vi "Open measure - MAIN.vi"() -> ()   [LabVIEW 2019]
uses:
  OPEN STATUS.ctl
  Open measure - global.vi
panel:
  in  "Normalize":bool
  in  "Remove baseline":bool
  in  "Export image":bool
  out "Phase":cluster{"all rows":dbl[], "all rows":dbl[]}[](graph)
  in  "Add Button":bool
  in  "Clear":bool
  in  "Stop Button":bool
  in  "Plot_name (if only one)":string
  out "Amplitude":cluster{"all rows":dbl[], "all rows":dbl[]}[](graph)
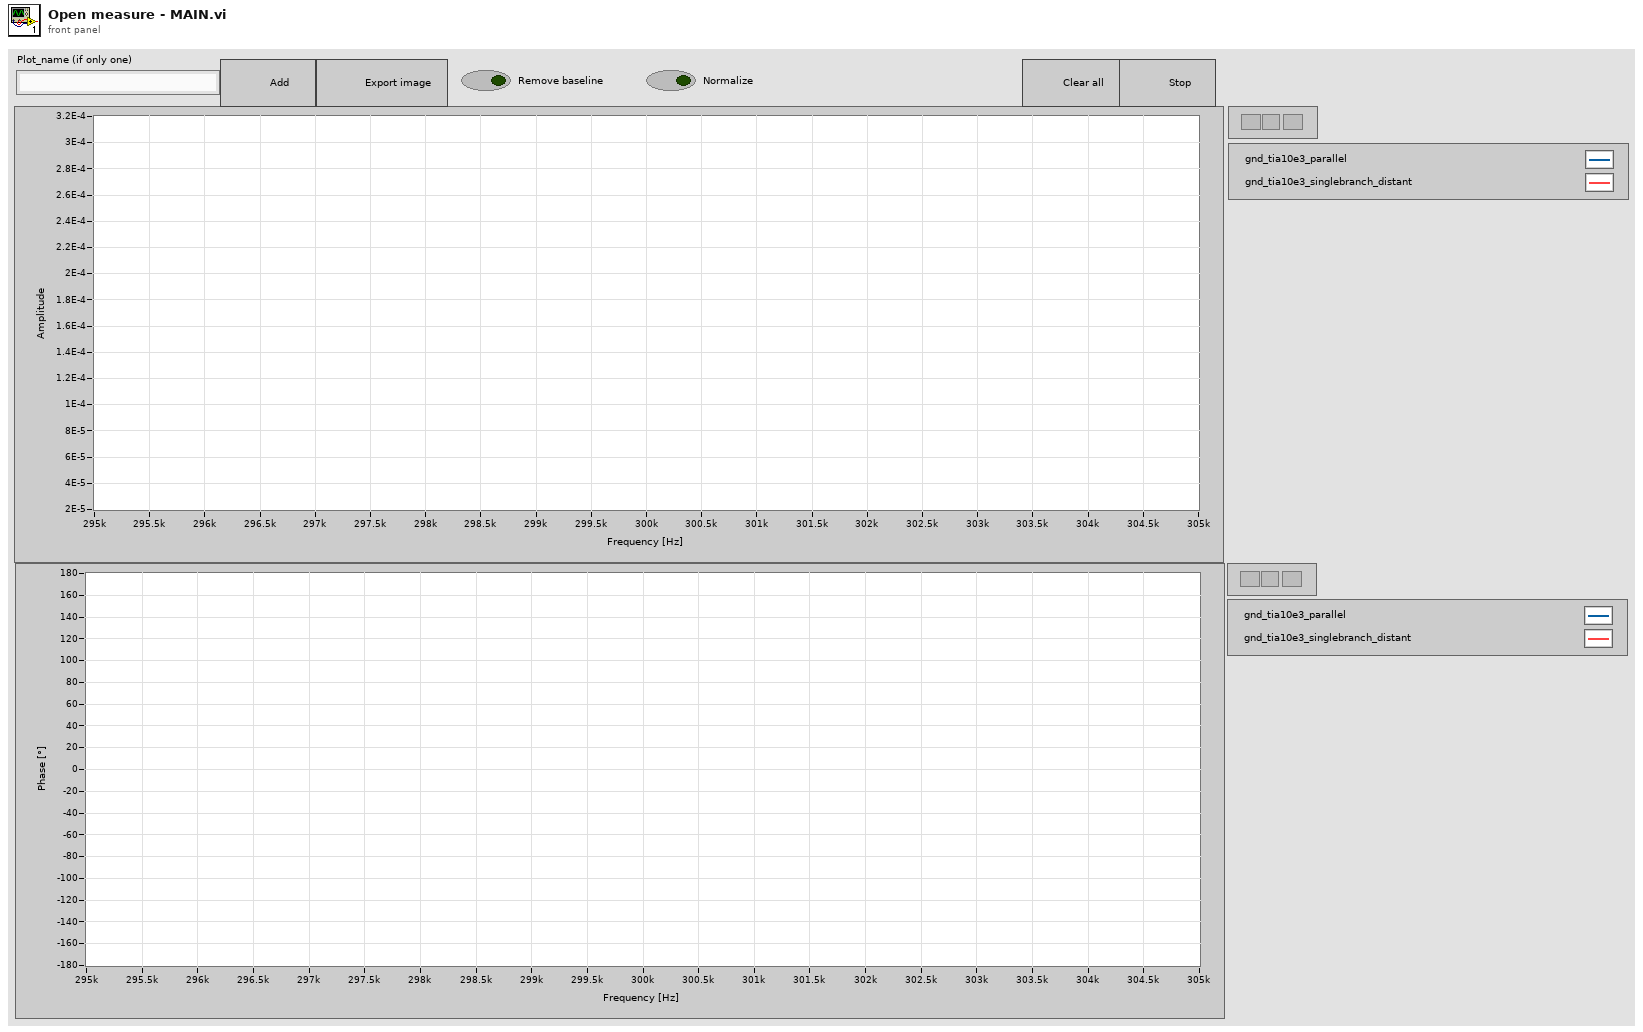
[diagram p1: front panel]
types:
  T1 = typedef "OPEN STATUS.ctl" = cluster{enum16{"Idle", "Stop", "Clear", "Export", "Add"}, "element data type":variant}
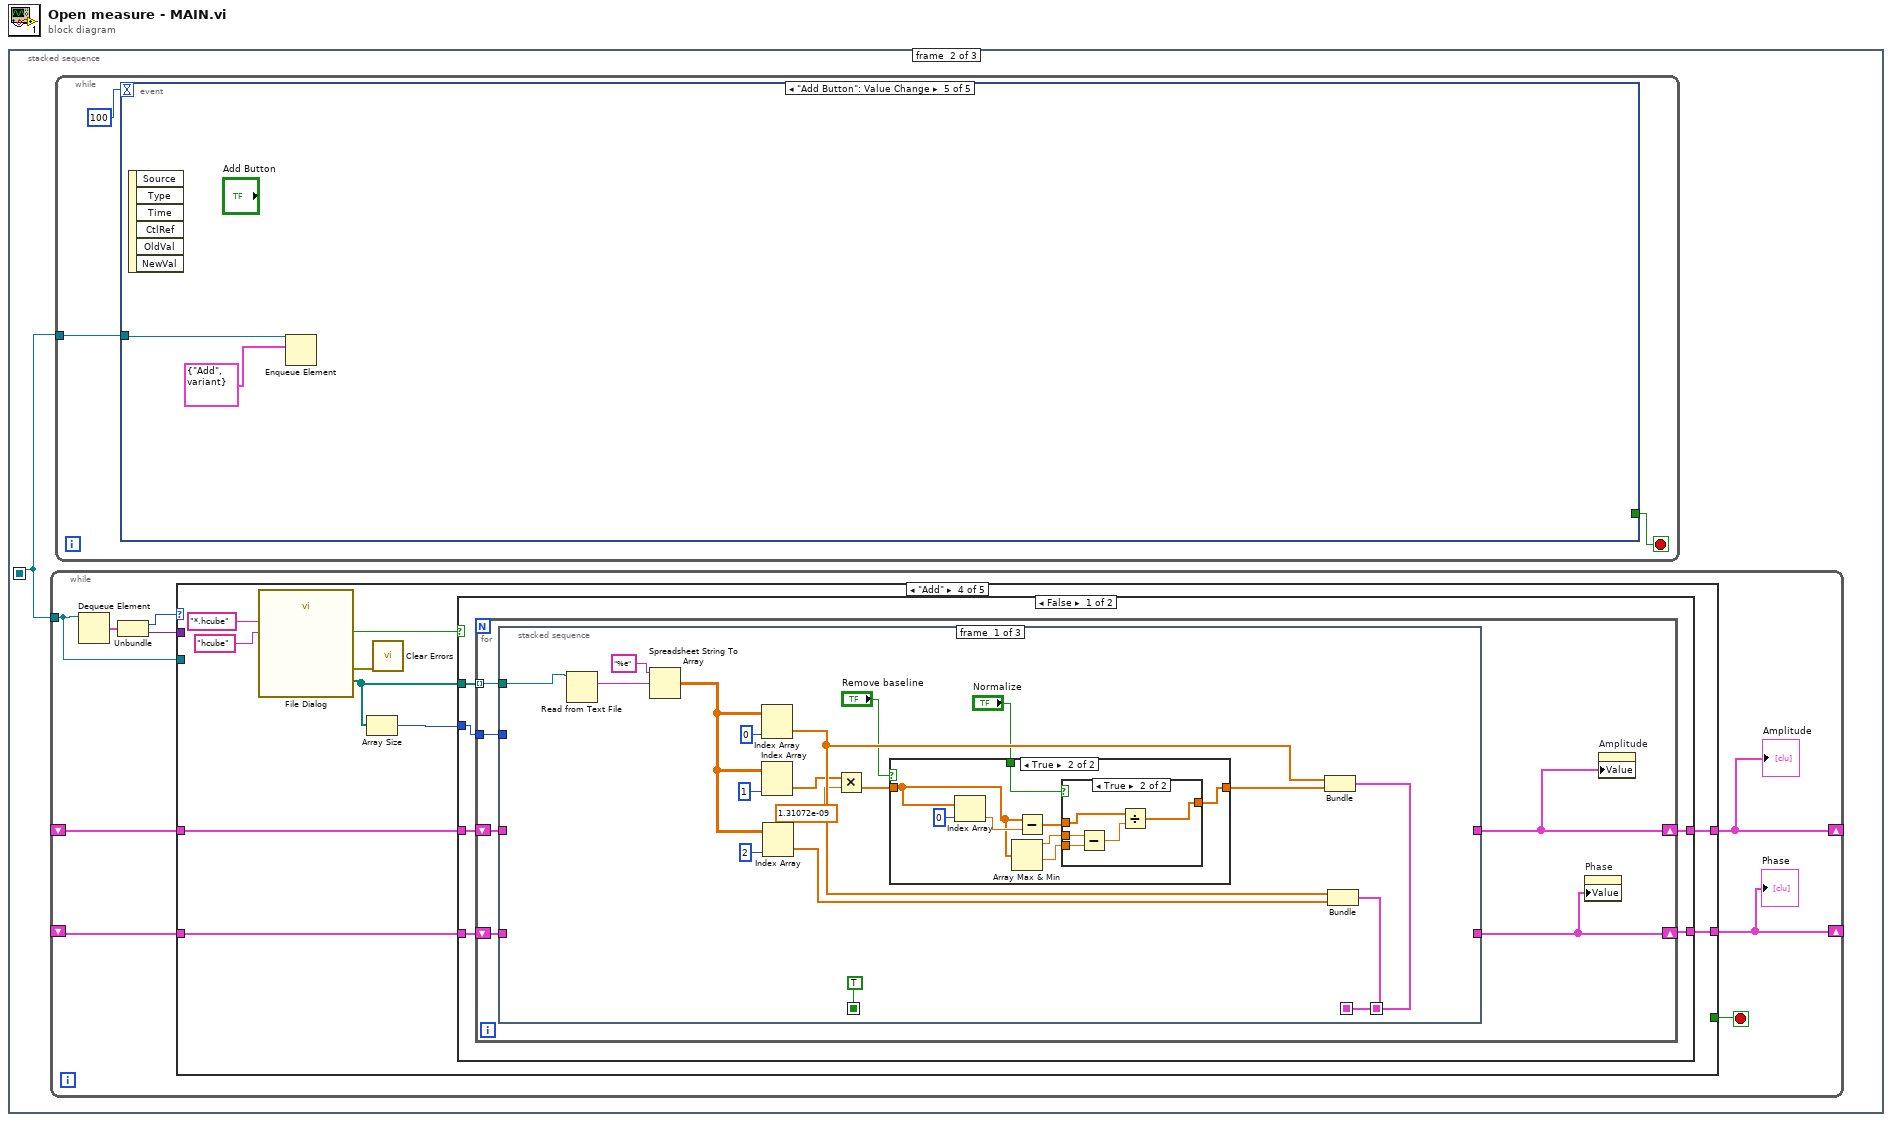
[diagram p0: block diagram]
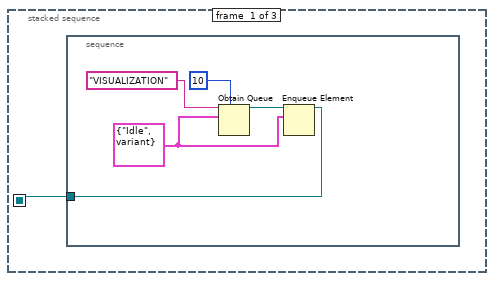
[diagram p2: hidden frame]
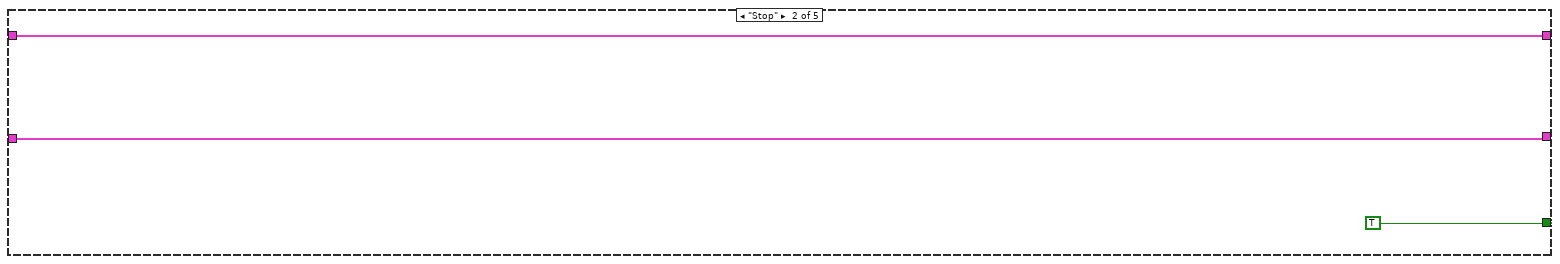
[diagram p4: hidden frame]
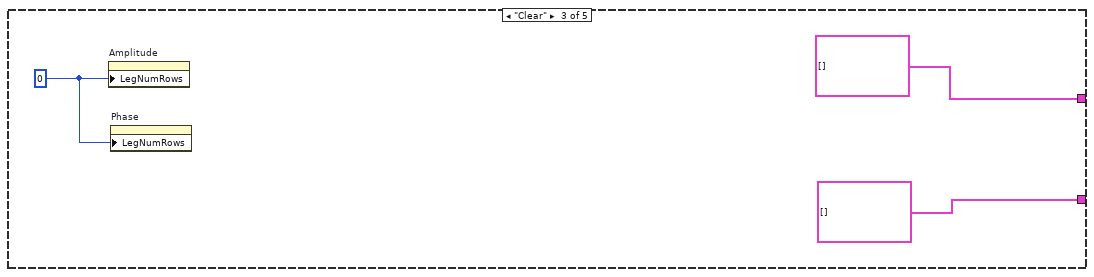
[diagram p5: hidden frame]
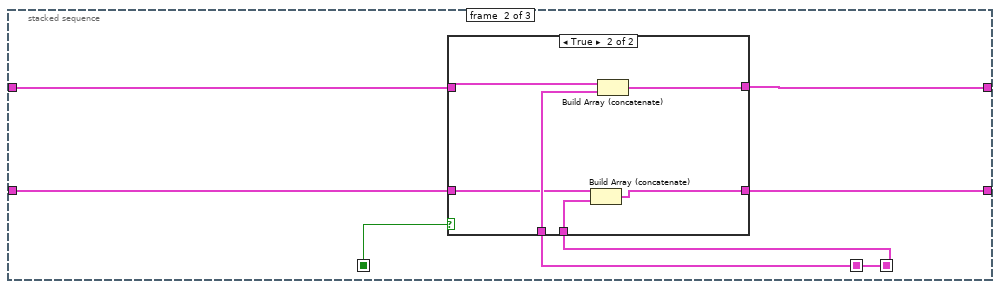
[diagram p8: hidden frame]
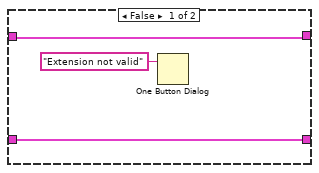
[diagram p9: hidden frame]
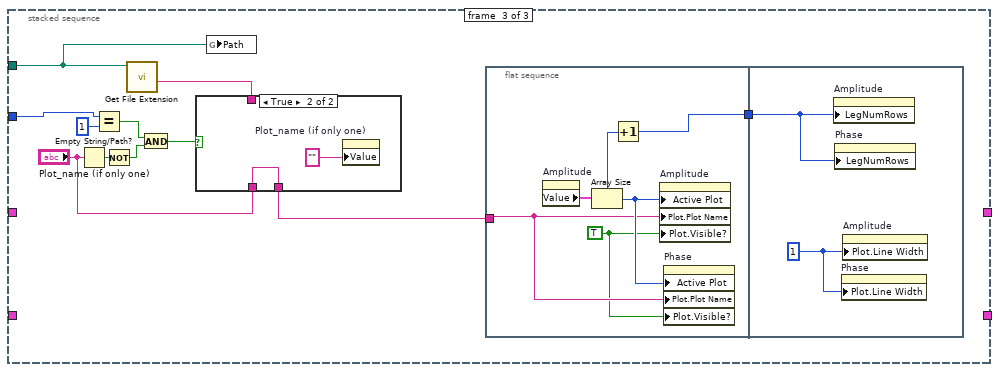
[diagram p10: hidden frame]
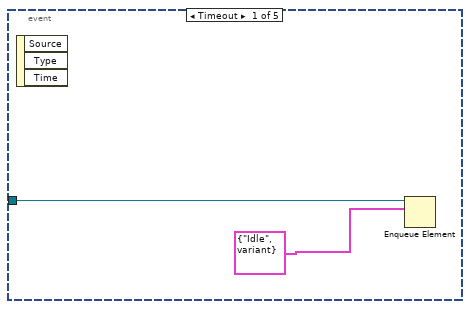
[diagram p14: hidden frame]
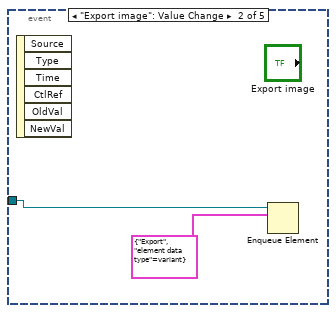
[diagram p15: hidden frame]
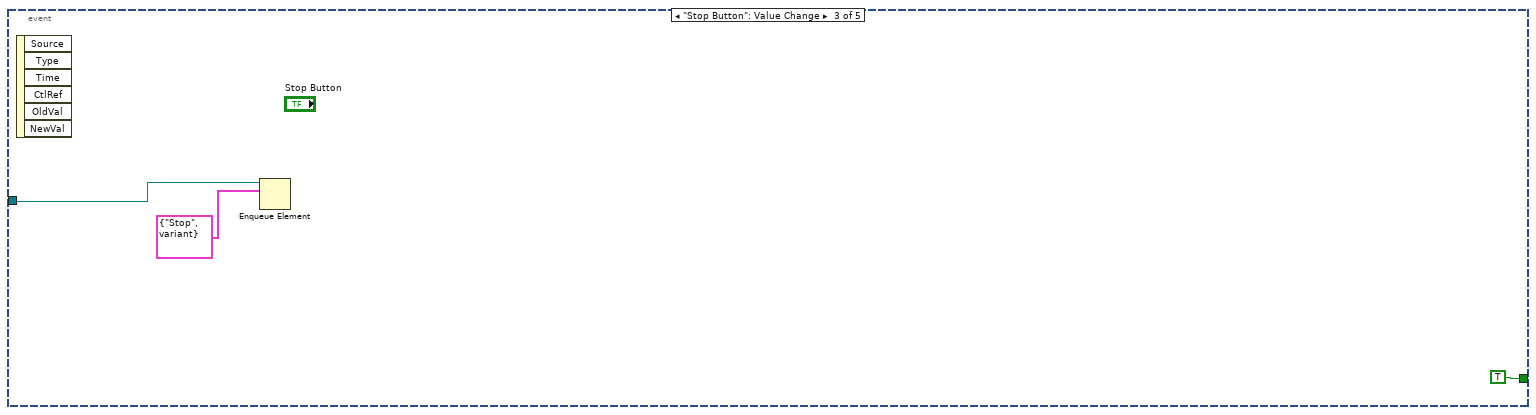
[diagram p16: hidden frame]
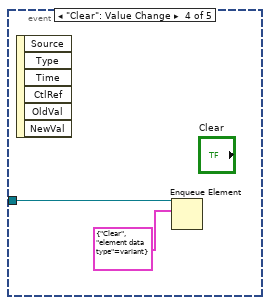
[diagram p17: hidden frame]
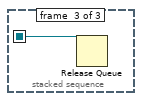
[diagram p18: hidden frame]
diagram:
  n1 = stacked-sequence {
    seq-local: [w1 _ _] -> [_ w7 w135]
    frame #0 {
      n2 = stacked-sequence {
        tunnel: [w3] -> w1
        frame #0 {
          w2 = T1 {enum."Idle", "element data type"=variant} ("Cluster")
          n3 = Obtain Queue(max queue size (-1, unlimited)=10, name (unnamed)="VISUALIZATION", element data type=w2) -> (queue out=w4:refnum<queue>)  [unwired: 2 in, 2 out]
          n4 = Enqueue Element(queue=w4, element=w2) -> (queue out=w3:refnum<queue>)  [unwired: 2 in, 2 out]
        }
      }
    }
    frame #1 {
      n5 = while {
        tunnel: w7 -> [w14]
        shift-right: [w11] -> _
        shift-left: _ -> [w10]
        shift-right: [w8] -> _
        shift-left: _ -> [w9]
        stop <- w12 stop-if-true
        n6 = Dequeue Element(queue=w14) -> (element=w16:T1)  [unwired: 2 in, 3 out]
        n7 = Unbundle(w16) -> (w13:enum16{"Idle", "Stop", "Clear", "Export", "Add"}, "element data type"=w15:variant)
        n8 = case shown="\"Add\"" w13 {
          tunnel: w15 -> [_ _ _ _ _]
          tunnel: w14 -> [_ _ _ _ _]
          tunnel: [_ TRUE _ _ _] -> w12
          tunnel: [w18 w20 cluster{"all rows":dbl[], "all rows":dbl[]}[] [] w33 w120] -> w11
          tunnel: w10 -> [w18 w20 _ w34 w120]
          tunnel: [w17 w19 cluster{"all rows":dbl[], "all rows":dbl[]}[] [] w26 w119] -> w8
          tunnel: w9 -> [w17 w19 _ w25 w119]
          frame "Idle", Default {
          }
          frame "Stop" {
          }
          frame "Clear" {
            w22 = u32 0 ("Legend:Size:Height")
            n9 = property on="Amplitude" class="XYGraph (strict)"("LegNumRows"=w22) -> ()  [unwired: 2 in, 2 out]
            n10 = property on="Phase" class="XYGraph (strict)"("LegNumRows"=w22) -> ()  [unwired: 2 in, 2 out]
          }
          frame "Add" {
            n11 = call "File Dialog"("pattern (all files)"="*.hcube" ("pattern label"), "pattern label"="hcube") -> ("selected paths"=w32:path[], "cancelled"=w30:bool, "error out"=w29:errorcluster)  [unwired: 10 in, 1 out]
            n12 = Array Size(array=w32) -> (size(s)=w31:i32)
            n13 = call <vilib>:"Clear Errors.vi"("error in (no error)"=w29) -> ()  [unwired: 5 in, 2 out]
            n14 = case shown="False" w30 {
              tunnel: w34 -> [w40 w118]
              tunnel: [w39 w118] -> w33
              tunnel: w32 -> [w38 _]
              tunnel: w31 -> [w37 _]
              tunnel: [w36 w117] -> w26
              tunnel: w25 -> [w35 w117]
              frame False {
                n15 = for {
                  tunnel: w38 -> [w45] mode=indexing
                  tunnel: w37 -> [w44]
                  shift-right: [w43] -> w39
                  shift-left: w40 -> [w46]
                  shift-right: [w41] -> w36
                  shift-left: w35 -> [w42]
                  n16 = stacked-sequence {
                    seq-local: [TRUE _ _] -> [_ w86 _]
                    seq-local: [w63 _ _] -> [_ w84 _]
                    seq-local: [w53 _ _] -> [_ w80 _]
                    tunnel: w46 -> [_ w85 _]
                    tunnel: [_ w83 _] -> w43
                    tunnel: w45 -> [w62 _ w96]
                    tunnel: w44 -> [_ _ w99]
                    tunnel: w42 -> [_ w82 _]
                    tunnel: [_ w81 _] -> w41
                    frame #0 {
                      n17 = Read from Text File(file (use dialog)=w62) -> (text=w61:string)  [unwired: 3 in, 3 out]
                      n18 = Spreadsheet String To Array(format string="%e", spreadsheet string=w61) -> (array=w56:dbl[][])  [unwired: 2 in]
                      n19 = Index Array(array=w56, index (col)=0 ("disabled index (col)")) -> (element=w54:dbl[])  [unwired: 1 in]
                      n20 = Index Array(array=w56, index (col)=1 ("disabled index (col)")) -> (element=w52:dbl[])  [unwired: 1 in]
                      n21 = Index Array(array=w56, index (col)=2 ("disabled index (col)")) -> (element=w55:dbl[])  [unwired: 1 in]
                      n22 = Multiply(x=w52, y=1.31072e-09) -> (x*y=w48:dbl[])
                      n23 = case shown="True" "Remove baseline" {
                        tunnel: w48 -> [w65 w69]
                        tunnel: [w65 w70] -> w51
                        tunnel: "Normalize" -> [_ w71]
                        frame False {
                        }
                        frame True {
                          n24 = Index Array(array=w69, index=0) -> (element=w72:dbl)
                          n25 = Array Max & Min(array=w69) -> (max value=w68:dbl, min value=w67:dbl)  [unwired: 2 out]
                          n26 = Subtract(x=w69, y=w72) -> (x-y=w66:dbl[])
                          n27 = case shown="True" w71 {
                            tunnel: [w74 w75] -> w70
                            tunnel: w66 -> [w74 w76]
                            tunnel: w68 -> [_ w78]
                            tunnel: w67 -> [_ w77]
                            frame False {
                            }
                            frame True {
                              n28 = Subtract(x=w78, y=w77) -> (x-y=w79:dbl)
                              n29 = Divide(x=w76, y=w79) -> (x/y=w75:dbl[])
                            }
                          }
                        }
                      }
                      n30 = Bundle(w54, w51) -> (w63:cluster{dbl[], dbl[]})  [unwired: 1 in]
                      n31 = Bundle(w54, w55) -> (w53:cluster{dbl[], dbl[]})  [unwired: 1 in]
                    }
                    frame #1 {
                      n32 = case shown="True" w86 {
                        tunnel: w85 -> [w89 w95]
                        tunnel: w84 -> [_ w94]
                        tunnel: [w89 w93] -> w83
                        tunnel: w82 -> [w87 w92]
                        tunnel: [w87 w91] -> w81
                        tunnel: w80 -> [_ w90]
                        frame False {
                          n33 = One Button Dialog(message="Extension not valid") -> ()  [unwired: 1 in, 1 out]
                        }
                        frame True {
                          n34 = Build Array (concatenate)(w92, w90) -> (w91:cluster{"all rows":dbl[], "all rows":dbl[]}[])
                          n35 = Build Array (concatenate)(w95, w94) -> (w93:cluster{"all rows":dbl[], "all rows":dbl[]}[])
                        }
                      }
                    }
                    frame #2 {
                      n36 = Empty String/Path?(string/path="Plot_name (if only one)") -> (empty?=w105:bool)
                      n37 = Equal?(x=w99, y=1) -> (x = y?=w103:bool)
                      n38 = Not(x=w105) -> (.not. x?=w104:bool)
                      n39 = call <vilib>:"Get File Extension.vi"("file"=w96) -> ("filename without extension"=w97:string)  [unwired: 6 in, 4 out]
                      n40 = And(x=w103, y=w104) -> (x .and. y?=w102:bool)
                      n41 = case shown="True" w102 {
                        tunnel: [w107 w109] -> w101
                        tunnel: "Plot_name (if only one)" -> [_ w109]
                        tunnel: w97 -> [w107 _]
                        frame False {
                        }
                        frame True {
                          n42 = property on="Plot_name (if only one)" class="Str"("Value"="" ("Plot_name (if only one)")) -> ()  [unwired: 2 in, 2 out]
                        }
                      }
                      n43 = global write "Open measure - global.vi" "Path"(w96) -> ()
                      n44 = flat-sequence {
                        tunnel: w101 -> [w111]
                        tunnel: [w113] -> w98
                        tunnel: w98 -> [w115]
                        frame #0 {
                          w110 = TRUE ("Plot.Visible")
                          n45 = property on="Amplitude" class="XYGraph (strict)"() -> ("Value"=w114:cluster{"all rows":dbl[], "all rows":dbl[]}[])  [unwired: 2 in, 2 out]
                          n46 = Array Size(array=w114) -> (size(s)=w112:i32)
                          n47 = Increment(x=w112) -> (x+1=w113:i32)
                          n48 = property on="Amplitude" class="XYGraph (strict)"("Active Plot"=w112, "Plot.Plot Name"=w111, "Plot.Visible?"=w110) -> ()  [unwired: 2 in, 2 out]
                          n49 = property on="Phase" class="XYGraph (strict)"("Active Plot"=w112, "Plot.Plot Name"=w111, "Plot.Visible?"=w110) -> ()  [unwired: 2 in, 2 out]
                        }
                        frame #1 {
                          w116 = u8 1 ("Plot.Line Width")
                          n50 = property on="Amplitude" class="XYGraph (strict)"("LegNumRows"=w115) -> ()  [unwired: 2 in, 2 out]
                          n51 = property on="Phase" class="XYGraph (strict)"("LegNumRows"=w115) -> ()  [unwired: 2 in, 2 out]
                          n52 = property on="Phase" class="XYGraph (strict)"("Plot.Line Width"=w116) -> ()  [unwired: 2 in, 2 out]
                          n53 = property on="Amplitude" class="XYGraph (strict)"("Plot.Line Width"=w116) -> ()  [unwired: 2 in, 2 out]
                        }
                      }
                    }
                  }
                  n54 = property on="Phase" class="XYGraph (strict)"("Value"=w41) -> ()  [unwired: 2 in, 2 out]
                  n55 = property on="Amplitude" class="XYGraph (strict)"("Value"=w43) -> ()  [unwired: 2 in, 2 out]
                }
              }
              frame True {
              }
            }
          }
          frame "Export" {
          }
        }
        "Amplitude" <- w11
        "Phase" <- w8
      }
      n56 = while {
        tunnel: w7 -> [w122]
        stop <- w121 stop-if-true
        n57 = event shown="[4] \"Add Button\": Value Change" {
          selector: _ -> [_ _ _ _ _]
          dyn-events: _ -> [_ _ _ _ _]
          timeout: 100 -> [_ _ _ _ _]
          tunnel: w122 -> [w125 w127 w129 w132 w134]
          tunnel: [_ _ TRUE _ _] -> w121
          event Timeout {
            n58 = event-data() -> ()  [unwired: 1 in, 3 out]
            n59 = Enqueue Element(queue=w125, element=T1 {enum."Idle", "element data type"=variant} ("Cluster")) -> ()  [unwired: 2 in, 3 out]
          }
          event "Export image": Value Change {
            n60 = event-data() -> ()  [unwired: 1 in, 6 out]
            n61 = Enqueue Element(queue=w127, element=T1 {enum."Export", "element data type"=variant} ("Cluster")) -> ()  [unwired: 2 in, 3 out]
          }
          event "Stop Button": Value Change {
            n62 = event-data() -> ()  [unwired: 1 in, 6 out]
            n63 = Enqueue Element(queue=w129, element=T1 {enum."Stop", "element data type"=variant} ("Cluster")) -> ()  [unwired: 2 in, 3 out]
          }
          event "Clear": Value Change {
            n64 = event-data() -> ()  [unwired: 1 in, 6 out]
            n65 = Enqueue Element(queue=w132, element=T1 {enum."Clear", "element data type"=variant} ("Cluster")) -> ()  [unwired: 2 in, 3 out]
          }
          event "Add Button": Value Change {
            n66 = event-data() -> ()  [unwired: 1 in, 6 out]
            n67 = Enqueue Element(queue=w134, element=T1 {enum."Add", "element data type"=variant} ("Cluster")) -> ()  [unwired: 2 in, 3 out]
          }
        }
      }
    }
    frame #2 {
      n68 = Release Queue(queue=w135) -> ()  [unwired: 2 in, 3 out]
    }
  }
